vi "CAN Frame to std frm.vi"(1 "Channel":i32, 3 "CAN Frame":T2(array[cluster])) -> (0 "CAN Std Frm":T1[](array[typedef]) {"Direction" items=["Tx", "Rx"]; "CANType" items=["CAN", "CANFD", "CANFD加速"]})   [LabVIEW 2018, in "CAN FD.lvlib"]
uses:
  CAN FD.lvlib
  Typedef/CAN Data.ctl
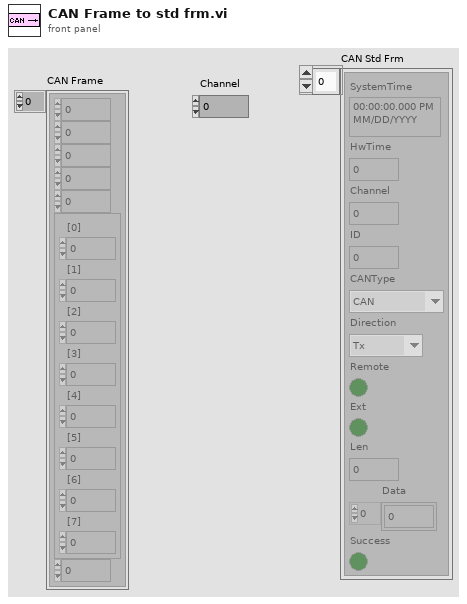
[diagram p1: front panel]
types:
  T1 = typedef "CAN FD.lvlib/CAN Data.ctl" = cluster{"SystemTime":timestamp, "HwTime":dbl, "Channel":u8, "ID":u32, "CANType":i16, "Direction":i16, "Remote":bool, "Ext":bool, "Len":u8, "Data":u8[], "Success":bool}
  T2 = cluster{u32, u8, u8, u8, u8, cluster{"[0]":u8, "[1]":u8, "[2]":u8, "[3]":u8, "[4]":u8, "[5]":u8, "[6]":u8, "[7]":u8}, u64}[]
  T3 = cluster{"[0]":u8, "[1]":u8, "[2]":u8, "[3]":u8, "[4]":u8, "[5]":u8, "[6]":u8, "[7]":u8}
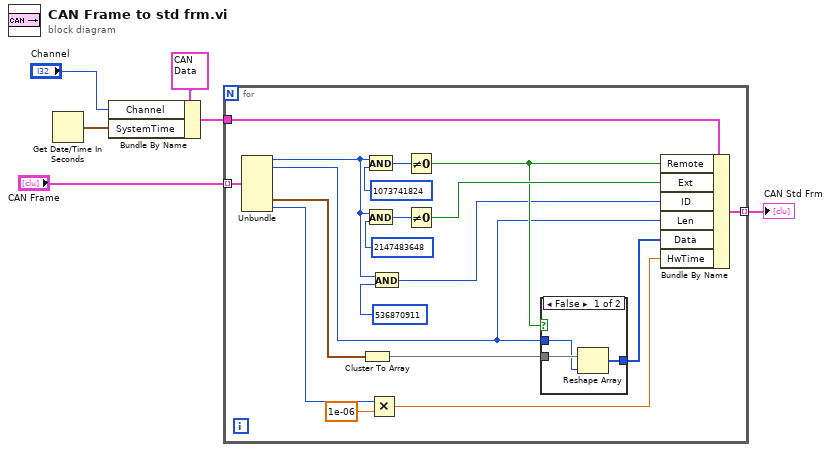
[diagram p0: block diagram]
diagram:
  n1 = Get Date/Time In Seconds() -> (seconds since 1Jan1904=w4:timestamp)
  n2 = Bundle By Name(cluster=T1 {"SystemTime"=timestamp(0 s since 1904-01-01), "HwTime"=0.0, "Channel"=0, "ID"=0, "CANType"=0, "Direction"=1, "Remote"=FALSE, "Ext"=FALSE, "Len"=0, "Data"=[], "Success"=FALSE} ("Data"), "Channel"="Channel", "SystemTime"=w4) -> (w3:T1)
  n3 = for {
    tunnel: "CAN Frame" -> [w17] mode=indexing
    tunnel: w3 -> [w16]
    tunnel: [w11] -> w2 mode=indexing
    n4 = Unbundle(w17) -> (w20:u32, w7:u8, w19:T3, w10:u64)  [unwired: 3 out]
    n5 = Cluster To Array(cluster=w19) -> (array=w18:u8[])
    n6 = And(x=w20, y=u32 1073741824) -> (x .and. y?=w21:u32)
    n7 = And(x=w20, y=u32 2147483648) -> (x .and. y?=w22:u32)
    n8 = Multiply(x=w10, y=1e-06) -> (x*y=w8:dbl)
    n9 = And(x=w20, y=u32 536870911) -> (x .and. y?=w12:u32)
    n10 = Not Equal To 0?(x=w21) -> (x != 0?=w14:bool)
    n11 = Not Equal To 0?(x=w22) -> (x != 0?=w15:bool)
    n12 = case shown="False" w14 {
      tunnel: [w26 _] -> w13
      tunnel: w18 -> [w28 _]
      tunnel: w7 -> [w27 _]
      frame False {
        n13 = Reshape Array(w28, w27) -> (w26:u8[])
      }
      frame True {
      }
    }
    n14 = Bundle By Name(cluster=w16, "Remote"=w14, "Ext"=w15, "ID"=w12, "Len"=w7, "Data"=w13, "HwTime"=w8) -> (w11:T1)
  }
  "CAN Std Frm" <- w2
